vi "Event_RefNum_Simulation_Global.vi"(0 "menu":enum16{"set", "get", "delete"}(ring)=enum."get", 7 "FRC_Sim_Events in":refnum<user-event>, 11 "error in (no error)":errorcluster) -> (8 "FRC_Sim_Events out":refnum<user-event>, 15 "error out":errorcluster)   [LabVIEW 2017]
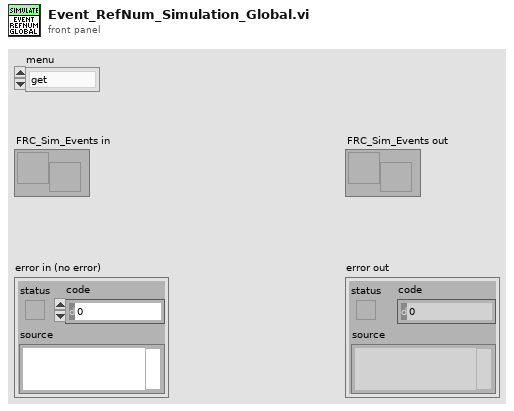
[diagram p1: front panel]
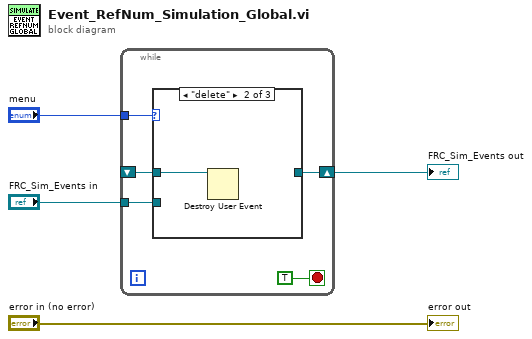
[diagram p0: block diagram]
diagram:
  n1 = while {
    tunnel: "menu" -> [w8]
    shift-right: [w6] -> w2
    shift-left: _ -> [w7]
    tunnel: "FRC_Sim_Events in" -> [w5]
    stop <- TRUE stop-if-true
    n2 = case shown="\"delete\"" w8 {
      tunnel: w7 -> [_ w11 w12]
      tunnel: [w10 _ w12] -> w6
      tunnel: w5 -> [w10 _ _]
      frame "set" {
      }
      frame "delete" {
        n3 = Destroy User Event(user event=w11) -> ()  [unwired: 1 in, 1 out]
      }
      frame "get", Default {
      }
    }
  }
  "FRC_Sim_Events out" <- w2
  "error out" <- "error in (no error)"
